vi "GetSurfaceInfo.vi"(8 "No Error":errorcluster, 11 "surface [SDL_Surface *]":i64) -> (0 "error out":errorcluster, 3 "Surface Info":T3 {"flag" items=["SDL_SURFACE_PREALLOCATED"=1, "SDL_SURFACE_LOCK_NEEDED"=2, "SDL_SURFACE_LOCKED"=4, "SDL_SURFACE_SIMD_ALIGNED"=8]})   [LabVIEW 2024, in "SDL3.lvlib" / "Surface.lvlib"]
doc: "<B>Summary</B>\nCreates a new surface identical to the existing surface.\n\n<B>Remarks</B>\nIf the original surface has alternate images, the new surface will have a reference to them as well.\n\nThe returned surface should be freed with SDL_DestroySurface()."
uses:
  Surface.lvlib
  SurfaceFlags--ring.ctl
  Pixels/PixelFormat--enum.ctl
  LV-Utilities/LV-Utilities.lvlib
  Pixels/Pixels.lvlib
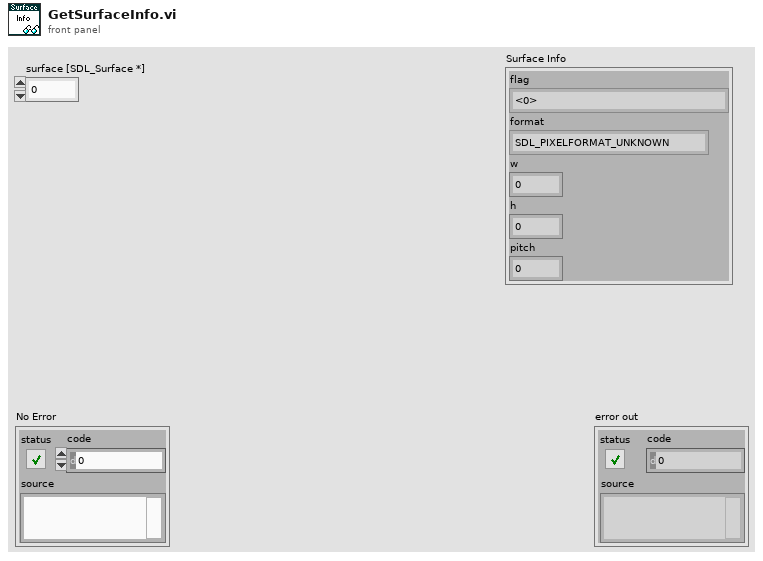
[diagram p1: front panel]
types:
  T1 = typedef "SDL3.lvlib/Surface.lvlib/SurfaceFlags--ring.ctl" = u32
  T2 = typedef "SDL3.lvlib/Pixels.lvlib/PixelFormat--enum.ctl" = enum32{"SDL_PIXELFORMAT_UNKNOWN", "SDL_PIXELFORMAT_INDEX1LSB", "SDL_PIXELFORMAT_INDEX1MSB", "SDL_PIXELFORMAT_INDEX2LSB", "SDL_PIXELFORMAT_INDEX2MSB", "SDL_PIXELFORMAT_INDEX4LSB", "SDL_PIXELFORMAT_INDEX4MSB", "SDL_PIXELFORMAT_INDEX8", "SDL_PIXELFORMAT_RGB332", "SDL_PIXELFORMAT_XRGB4444", "SDL_PIXELFORMAT_XBGR4444", "SDL_PIXELFORMAT_XRGB1555", "SDL_PIXELFORMAT_XBGR1555", "SDL_PIXELFORMAT_ARGB4444", "SDL_PIXELFORMAT_RGBA4444", "SDL_PIXELFORMAT_ABGR4444", "SDL_PIXELFORMAT_BGRA4444", "SDL_PIXELFORMAT_ARGB1555", "SDL_PIXELFORMAT_RGBA5551", "SDL_PIXELFORMAT_ABGR1555", "SDL_PIXELFORMAT_BGRA5551", "SDL_PIXELFORMAT_RGB565", "SDL_PIXELFORMAT_BGR565", "SDL_PIXELFORMAT_RGB24", "SDL_PIXELFORMAT_BGR24", "SDL_PIXELFORMAT_XRGB8888", "SDL_PIXELFORMAT_RGBX8888", "SDL_PIXELFORMAT_XBGR8888", "SDL_PIXELFORMAT_BGRX8888", "SDL_PIXELFORMAT_ARGB8888", "SDL_PIXELFORMAT_RGBA8888", "SDL_PIXELFORMAT_ABGR8888", "SDL_PIXELFORMAT_BGRA8888", "SDL_PIXELFORMAT_XRGB2101010", "SDL_PIXELFORMAT_XBGR2101010", "SDL_PIXELFORMAT_ARGB2101010", "SDL_PIXELFORMAT_ABGR2101010", "SDL_PIXELFORMAT_RGB48", "SDL_PIXELFORMAT_BGR48", "SDL_PIXELFORMAT_RGBA64", "SDL_PIXELFORMAT_ARGB64", "SDL_PIXELFORMAT_BGRA64", "SDL_PIXELFORMAT_ABGR64", "SDL_PIXELFORMAT_RGB48_FLOAT", "SDL_PIXELFORMAT_BGR48_FLOAT", "SDL_PIXELFORMAT_RGBA64_FLOAT", "SDL_PIXELFORMAT_ARGB64_FLOAT", "SDL_PIXELFORMAT_BGRA64_FLOAT", "SDL_PIXELFORMAT_ABGR64_FLOAT", "SDL_PIXELFORMAT_RGB96_FLOAT", "SDL_PIXELFORMAT_BGR96_FLOAT", "SDL_PIXELFORMAT_RGBA128_FLOAT", "SDL_PIXELFORMAT_ARGB128_FLOAT", "SDL_PIXELFORMAT_BGRA128_FLOAT", "SDL_PIXELFORMAT_ABGR128_FLOAT", "SDL_PIXELFORMAT_YV12", "SDL_PIXELFORMAT_IYUV", "SDL_PIXELFORMAT_YUY2", "SDL_PIXELFORMAT_UYVY", "SDL_PIXELFORMAT_YVYU", "SDL_PIXELFORMAT_NV12", "SDL_PIXELFORMAT_NV21", "SDL_PIXELFORMAT_P010", "SDL_PIXELFORMAT_EXTERNAL_OES"}
  T3 = cluster{"flag":T1, "format":T2, "w":i32, "h":i32, "pitch":i32}
  T4 = cluster{"flag":T1, "format":u32, "w":i32, "h":i32, "pitch":i32}
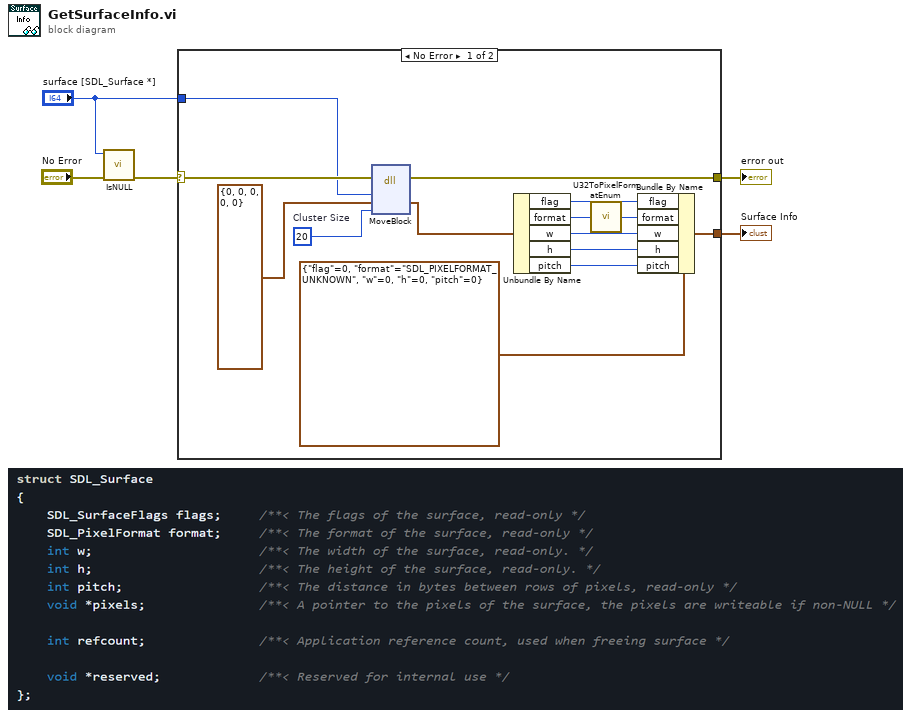
[diagram p0: block diagram]
diagram:
  n1 = call "IsNULL.vi"("error in (no error)"="No Error", "ptr"="surface [SDL_Surface *]") -> ("error out"=w3:errorcluster)  [unwired: 9 in]
  n2 = case shown="No Error" w3 {
    selector: w3 -> [w19 w20]
    tunnel: [w14 w20] -> w4
    tunnel: "surface [SDL_Surface *]" -> [w16 _]
    tunnel: [w6 _] -> w1
    frame No Error {
      w17 = 20  # Cluster Size
      n3 = dll-call lib="LabVIEW" fn="MoveBlock"(error in=w19, "Address"=w16, "Destination"=T4 {"flag"=0, "format"=0, "w"=0, "h"=0, "pitch"=0}, "Size"=w17) -> (error out=w14:errorcluster, "Destination"=w15:T4)  [unwired: 5 in, 1 out]
      n4 = Unbundle By Name(w15) -> ("flag"=w12:T1, "format"=w10:u32, "w"=w11:i32, "h"=w8:i32, "pitch"=w7:i32)
      n5 = call "U32ToPixelFormatEnum.vi"("pixel_format_integer"=w10) -> ("pixel_format_enum"=w9:T2)
      n6 = Bundle By Name(cluster=T3 {"flag"=0, "format"=enum."SDL_PIXELFORMAT_UNKNOWN", "w"=0, "h"=0, "pitch"=0}, "flag"=w12, "format"=w9, "w"=w11, "h"=w8, "pitch"=w7) -> (w6:T3)
    }
    frame Error {
    }
  }
  "error out" <- w4
  "Surface Info" <- w1
